vi "soft heap limit64.vi"(8 "error in (no error)":errorcluster, 11 "N":u64) -> (0 "error out":errorcluster, 3 "function return":u64)   [LabVIEW 2020, in "sqlite3.lvlib"]
uses:
  sqlite3.lvlib
  errstr.vi
  bin/sqlite3_64.dll
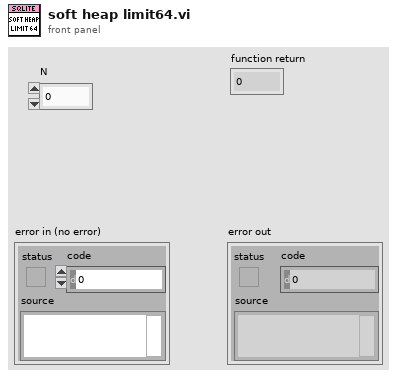
[diagram p1: front panel]
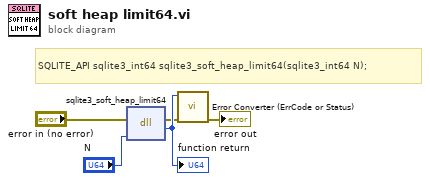
[diagram p0: block diagram]
diagram:
  # "SQLITE_API sqlite3_int64 sqlite3_soft_heap_limit64(sqlite3_int64 N);"
  n1 = dll-call lib="C:/Users/Fred.Guo/Desktop/Database-configuration/externals/sqlite3/Source/bin/sqlite3_*.*" fn="sqlite3_soft_heap_limit64"(error in="error in (no error)", "N"="N") -> (error out=w2:errorcluster, w5:u64)  [unwired: 3 in, 1 out]
  "function return" <- w5
  n2 = call "Error Converter (ErrCode or Status).vi"("error in (no error)"=w2, "error code"=w5) -> ("error out"=→"error out":errorcluster)  [unwired: 9 in]
